vi "DataObject_Create.vi"(0 "reference in":refnum<class "DataObject.lvclass">, 2 "StringRef":refnum<vi>, 5 "error in (no error)":errorcluster) -> (14 "reference out":refnum<class "DataObject.lvclass">, 19 "error out":errorcluster)   [LabVIEW 2020, in "DataObject.lvclass"]
uses:
  DataObject.lvclass
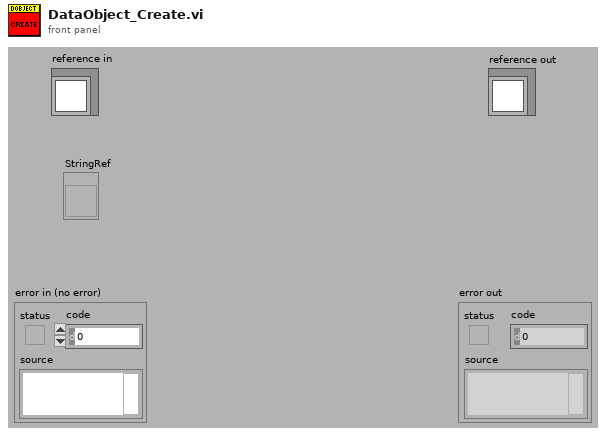
[diagram p1: front panel]
types:
  T1 = typedef "DataObject.lvclass/ObjectAttributes.ctl" = cluster{"StringRef":refnum<vi>}
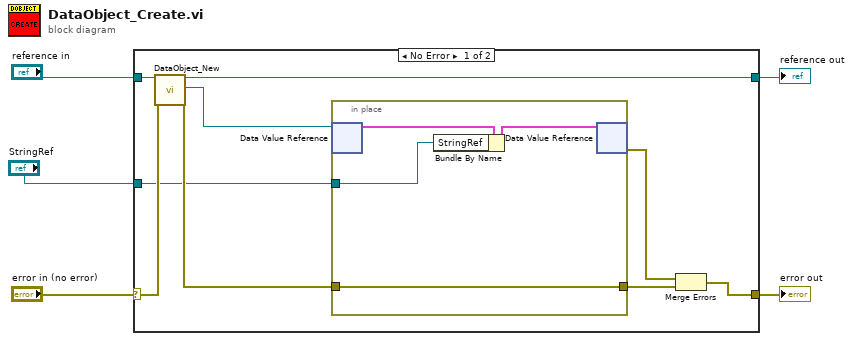
[diagram p0: block diagram]
diagram:
  n1 = case shown="No Error" "error in (no error)" {
    selector: "error in (no error)" -> [w13 w20]
    tunnel: [w10 w20] -> w4
    tunnel: "reference in" -> [w14 w19]
    tunnel: [w12 w19] -> w2
    tunnel: "StringRef" -> [w6 _]
    frame No Error {
      n2 = call "DataObject_New.vi"("reference in"=w14, "error in (no error)"=w13) -> ("reference out"=w12:refnum<class "DataObject.lvclass">, "DVRRefOut"=w9:refnum<data-value>, "error out"=w8:errorcluster)  [unwired: 14 in, 1 out]
      n3 = in-place {
        in-place-border: w8 -> [w18]
        in-place-border: [w18] -> w7
        in-place-border: w6 -> [w15]
        n4 = in-place-dvr #1(w9) -> (w17:T1)  [unwired: 1 out]
        n5 = Bundle By Name(cluster=w17, "StringRef"=w15) -> (w16:T1)
        n6 = in-place-dvr #1(w16) -> (w11:errorcluster)  [unwired: 1 out]
      }
      n7 = Merge Errors(w11, w7) -> (w10:errorcluster)
    }
    frame Error {
    }
  }
  "error out" <- w4
  "reference out" <- w2
